vi "Cmd.vi"(0 "reference":refnum<visa-resource-name>, 7 "Command String":string, 11 "String to receive":string) -> (4 "reference dup":refnum<visa-resource-name>, 8 "OK Done":bool, 15 "error out":errorcluster)   [LabVIEW 2011]
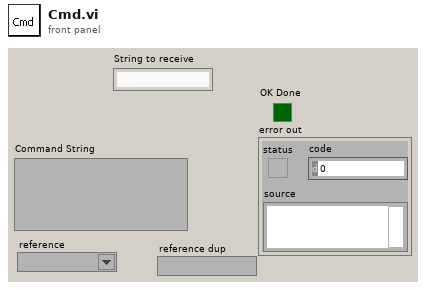
[diagram p1: front panel]
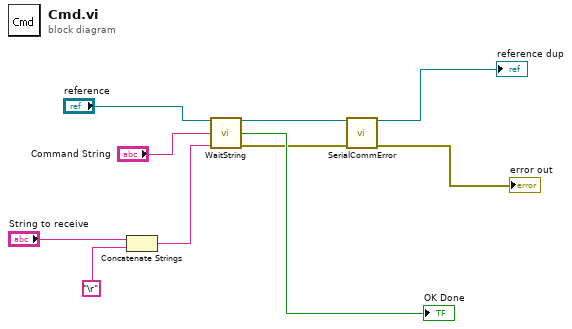
[diagram p0: block diagram]
diagram:
  n1 = Concatenate Strings("String to receive", "\r" ("string")) -> (w6:string)
  n2 = call "WaitString.vi"("reference"="reference", "String to Send"="Command String", "String to Receive"=w6) -> ("reference dup"=w4:refnum<visa-resource-name>, "OK Done"=→"OK Done":bool, "error out"=w3:errorcluster)  [unwired: 10 in]
  n3 = call "SerialCommError.vi"("VISA IN"=w4, "error IN"=w3) -> ("VISA OUT"=→"reference dup":refnum<visa-resource-name>, "error OUT"=→"error out":errorcluster)  [unwired: 11 in, 1 out]
